vi "UnMarshall.vi"(7 "Type":variant, 8 "error in (no error)":errorcluster, 10 "String":string, 11 "Serializer in":refnum<class "Serializer.lvclass">) -> (0 "error out":errorcluster, 2 "Variant":variant, 3 "Serializer out":refnum<class "Serializer.lvclass">)   [LabVIEW 2013, in "Serializer.lvclass"]
uses:
  Serializer.lvclass
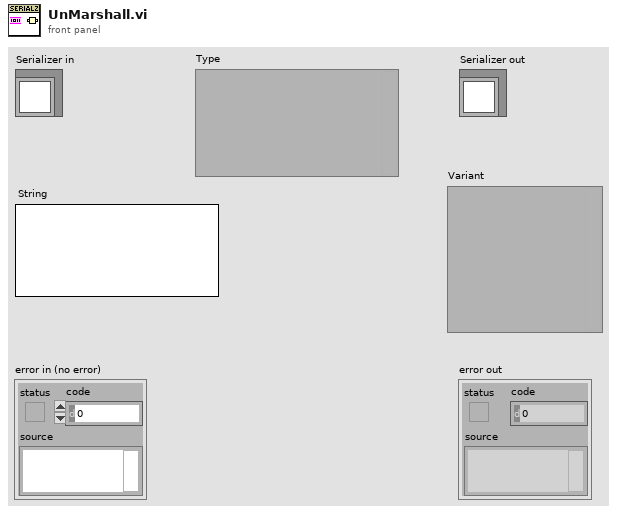
[diagram p1: front panel]
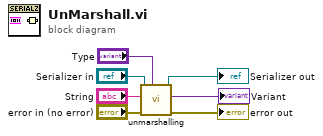
[diagram p0: block diagram]
diagram:
  n1 = call-dynamic "unmarshalling.vi"("Type"="Type", "error in (no error)"="error in (no error)", "String"="String", "Serializer in"="Serializer in") -> ("error out"=→"error out":errorcluster, "Variant"=→"Variant":variant, "Serializer out"=→"Serializer out":refnum<class "Serializer.lvclass">)  [unwired: 5 in]
